vi "Send Acknowledgement_SM.vi"(7 "Message Priority (Normal)":T2=enum."Normal", 8 "error in (no error)":errorcluster, 10 "Acknowledgement":T1, 11 "Message Enqueuer":refnum<class "Message Enqueuer.lvclass">) -> (0 "error out":errorcluster, 3 "Message Enqueuer out":refnum<class "Message Enqueuer.lvclass">)   [LabVIEW 2019, in "Acknowledgement_SM.lvclass"]
doc: "This VI sends the message to an actor."
uses:
  Acknowledgement_SM.lvclass
  <vilib>/ActorFramework/Message Enqueuer/Message Enqueuer.lvclass
  C:/Program Files/National Instruments/LabVIEW 2019/vi.lib/ActorFramework/Message/Message.lvclass
  <vilib>/ActorFramework/Message Enqueuer/Message Priority.ctl
  Common/Controls/Acknowledgement.ctl
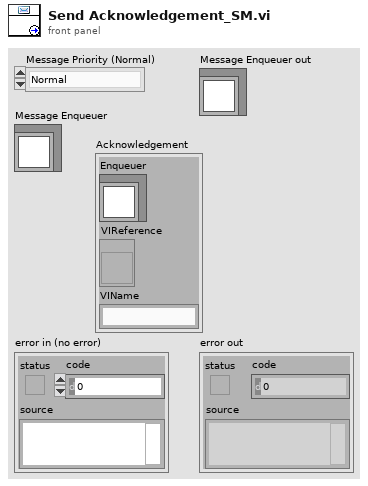
[diagram p1: front panel]
types:
  T1 = typedef "Acknowledgement.ctl" = cluster{"Enqueuer":refnum<class "Message Enqueuer.lvclass">, "VIReference":refnum<vi>, "VIName":string}
  T2 = typedef "Actor Framework.lvlib/Message Enqueuer.lvclass/Message Priority.ctl" = enum16{"Low", "Normal", "High"}
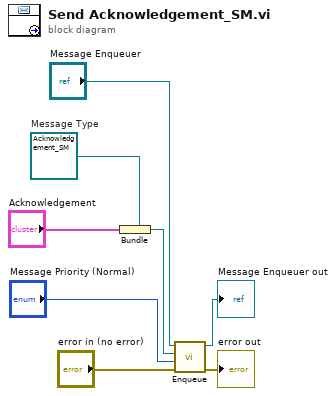
[diagram p0: block diagram]
diagram:
  w5 = refnum<class "Acknowledgement_SM.lvclass"> refnum  # Message Type
  n1 = Bundle(cluster=w5, "Acknowledgement") -> (w4:refnum<class "Acknowledgement_SM.lvclass">)
  n2 = call <vilib>:"Enqueue.vi"("error in (no error)"="error in (no error)", "Message Priority (Normal)"="Message Priority (Normal)", "Message"=w4, "Message Enqueuer in"="Message Enqueuer") -> ("error out"=→"error out":errorcluster, "Message Enqueuer out"=→"Message Enqueuer out":refnum<class "Message Enqueuer.lvclass">)  [unwired: 6 in]
